vi "contorno prueba.vi"() -> ()   [LabVIEW 2020]
uses:
  <vilib>/userDefined/High Color/IMAQdx.ctl
  <vilib>/vision/Management.llb/Cast Image 2 Method.ctl
  <vilib>/vision/Contour.llb/IMAQ Connect Range Setting.ctl
  <vilib>/vision/Contour.llb/IMAQ Contour Curve Extraction.ctl
  <vilib>/vision/driver/NI_Vision_Acquisition_Software.lvlib
  <vilib>/vision/NI_Vision_Development_Module.lvlib
panel:
  out "Image 2":T1(plugin-control)
  in  "y":u8
  out "Image":T1(plugin-control)
  out "new picture":picture
  in  "Session In":T2="cam1"
  in  "stop":bool
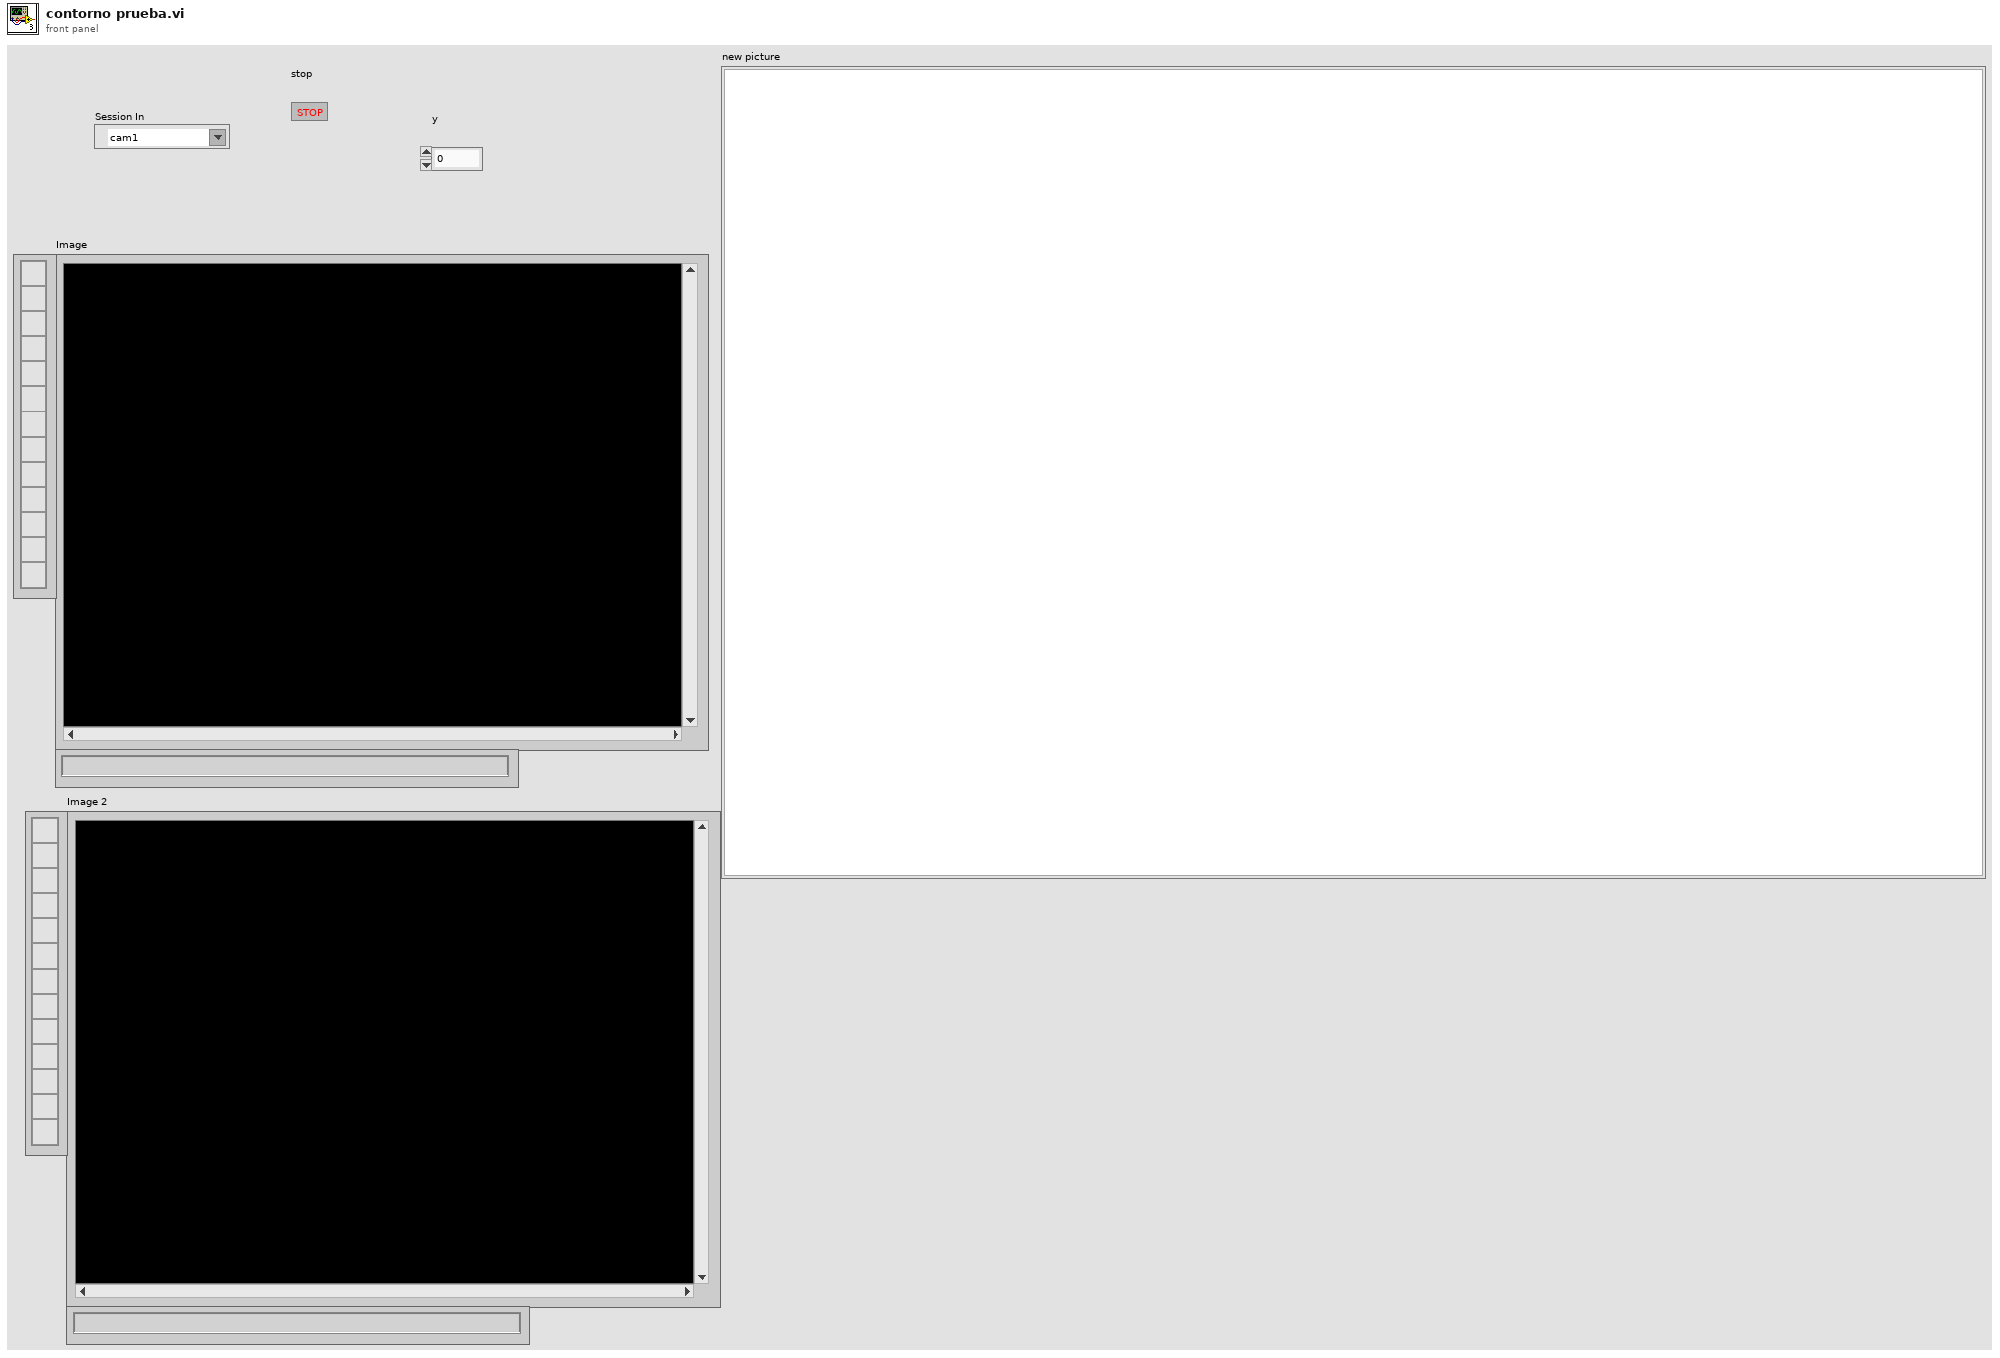
[diagram p1: front panel]
types:
  T1 = typedef "IMAQ Image.ctl" = refnum<image>
  T2 = typedef "IMAQdx.ctl" = refnum<k21>
  T3 = cluster{"Overlay?":bool, "Color":u32, "Width":u32, "Maintain Width?":bool}
  T4 = typedef "IMAQ Connect Range Setting.ctl" = cluster{"Match Constraints":u32, "Min":dbl, "Max":dbl}
  T5 = enum16{"Closest To Search Start", "Maximum Length", "Strongest Mean Gradient Change"}
  T6 = enum16{"Rect Left To Right", "Rect Right To Left", "Rect Top To Bottom", "Rect Bottom To Top", "Annulus Inner To Outer", "Annulus Outer To Inner", "Annulus Start Angle To End Angle", "Annulus End Angle To Start Angle"}
  T7 = typedef "IMAQ Contour Curve Extraction.ctl" = cluster{"Extraction Mode":u32, "Edge Threshold":i32, "Edge Filter Size":u32, "Min Length":i32, "Search Step Size":i32, "Max Endpoint Gap":i32, "Subpixel":bool}
  T8 = typedef "Image Type" = u32
  T9 = typedef "Cast Image 2 Method.ctl" = u32
  T10 = cluster{"Global Rectangle":i32[], "Contours":cluster{"Contour Type":u32, "ROI Type":u32, "Points":i32[]}[]}
  T11 = typedef "imagedata.ctl" = cluster{"image type":i32, "image depth":i32, "image":u8[], "mask":u8[], "colors":u32[], "Rectangle":cluster{"left":i16, "top":i16, "right":i16, "bottom":i16}}
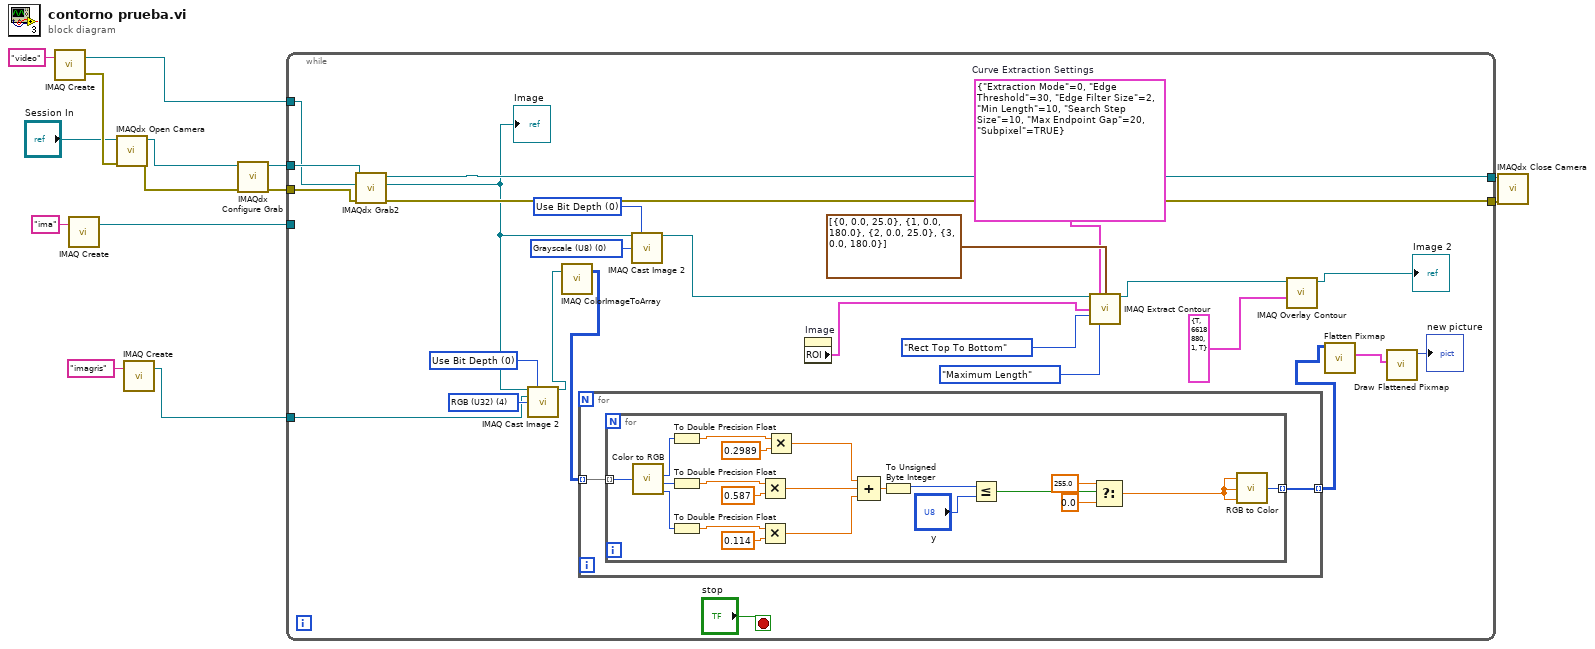
[diagram p0: block diagram]
diagram:
  n1 = call "IMAQ Create"("Image Name"="video") -> ("New Image"=w11:T1, "error out"=w14:errorcluster)  [unwired: 4 in]
  n2 = call "IMAQ Create"("Image Name"="ima") -> ("New Image"=w3:T1)  [unwired: 4 in, 1 out]
  n3 = call <vilib>:"IMAQdx Open Camera.vi"("error in"=w14, "Session In"="Session In") -> ("error out"=w7:errorcluster, "Session Out"=w13:T2)  [unwired: 8 in]
  n4 = call "IMAQ Create"("Image Name"="imagris") -> ("New Image"=w1:T1)  [unwired: 4 in, 1 out]
  n5 = call <vilib>:"IMAQdx Configure Grab.vi"("error in"=w7, "Session In"=w13) -> ("error out"=w8:errorcluster, "Session Out"=w12:T2)  [unwired: 8 in]
  n6 = while {
    tunnel: w12 -> [w40]
    tunnel: w11 -> [w39]
    tunnel: [w30] -> w10
    tunnel: [w29] -> w9
    tunnel: w8 -> [w37]
    tunnel: w3 -> [_]
    tunnel: w1 -> [w34]
    stop <- "stop" stop-if-true
    w20 = T7 {"Extraction Mode"=0, "Edge Threshold"=30, "Edge Filter Size"=2, "Min Length"=10, "Search Step Size"=10, "Max Endpoint Gap"=20, "Subpixel"=TRUE}  # Curve Extraction Settings
    w24 = T8 0 items=["Grayscale (U8)", "Grayscale (I16)", "Grayscale (SGL)", "Complex (CSG)", "RGB (U32)", "HSL (U32)", "RGB (U64)", "Grayscale (U16)"] ("Image Type")
    w25 = T9 0 items=["Use Bit Depth", "Shift", "Use Lookup Table"] ("Method")
    w35 = T9 0 items=["Use Bit Depth", "Shift", "Use Lookup Table"] ("Method")
    w36 = T8 4 items=["Grayscale (U8)", "Grayscale (I16)", "Grayscale (SGL)", "Complex (CSG)", "RGB (U32)", "HSL (U32)", "RGB (U64)", "Grayscale (U16)"] ("Image Type")
    n7 = call <vilib>:"IMAQdx Grab2.vi"("error in"=w37, "Image In"=w39, "Session In"=w40) -> ("error out"=w29:errorcluster, "Image Out"=w26:T1, "Session Out"=w30:T2)  [unwired: 5 in, 1 out]
    "Image" <- w26
    n8 = call "IMAQ Cast Image 2"("Image Src"=w26, "Method"=w35, "Image Dst"=w34, "Image Type"=w36) -> ("Image Dst Out"=w33:T1)  [unwired: 10 in, 1 out]
    n9 = call "IMAQ ColorImageToArray"("Image"=w33) -> ("Image Pixels (U32)"=w28:u32[][])  [unwired: 3 in, 2 out]
    n10 = for {
      tunnel: w28 -> [w42] mode=indexing
      tunnel: [w41] -> w27 mode=indexing
      n11 = for {
        tunnel: w42 -> [w63] mode=indexing
        tunnel: [w43] -> w41 mode=indexing
        n12 = call <vilib>:"Color to RGB.vi"("Color"=w63) -> ("R"=w62:u8, "G"=w61:u8, "B"=w60:u8)  [unwired: 1 out]
        n13 = To Double Precision Float(number=w62) -> (double precision float=w52:dbl)
        n14 = To Double Precision Float(number=w61) -> (double precision float=w51:dbl)
        n15 = To Double Precision Float(number=w60) -> (double precision float=w50:dbl)
        n16 = Multiply(x=w51, y=0.587) -> (x*y=w55:dbl)
        n17 = Multiply(x=w50, y=0.114) -> (x*y=w54:dbl)
        n18 = Multiply(x=w52, y=0.2989) -> (x*y=w56:dbl)
        n19 = Compound Arithmetic op=ADD(w56, w55, w54) -> (w53:dbl)
        n20 = To Unsigned Byte Integer(number=w53) -> (unsigned 8bit integer=w48:u8)
        n21 = Less Or Equal?(x=w48, y="y") -> (x <= y?=w47:bool)
        n22 = Select(t=255.0, s=w47, f=0.0) -> (s? t:f=w49:dbl)
        n23 = call <vilib>:"RGB to Color.vi"("B"=w49, "G"=w49, "R"=w49) -> ("Color"=w43:u32)
      }
    }
    n24 = call "IMAQ Cast Image 2"("Image Src"=w26, "Method"=w25, "Image Type"=w24) -> ("Image Dst Out"=w19:T1)  [unwired: 11 in, 1 out]
    n25 = property on="Image" class="ImageControl"() -> ("ROI"=w18:T10)  [unwired: 2 in, 2 out]
    n26 = call "IMAQ Extract Contour"("Source Image"=w19, "Curve Extraction"=w20, "ROI Descriptor"=w18, "Search Direction"=T6."Rect Top To Bottom", "Contour Selection"=T5."Maximum Length", "Curve Connection"=T4[] [{"Match Constraints"=0, "Min"=0.0, "Max"=25.0}, {"Match Constraints"=1, "Min"=0.0, "Max"=180.0}, {"Match Constraints"=2, "Min"=0.0, "Max"=25.0}, {"Match Constraints"=3, "Min"=0.0, "Max"=180.0}]) -> ("Source Image Out"=w16:T1)  [unwired: 2 in, 7 out]
    n27 = call "IMAQ Overlay Contour"("Contour Points Settings"=T3 {"Overlay?"=TRUE, "Color"=6618880, "Width"=1, "Maintain Width?"=TRUE}, "Image"=w16) -> ("Image Out"=→"Image 2":T1)  [unwired: 4 in, 5 out]
    n28 = call <vilib>:"Flatten Pixmap.vi"("24-bit pixmap"=w27) -> ("image data"=w32:T11)  [unwired: 10 in]
    n29 = call <vilib>:"Draw Flattened Pixmap.vi"("image data"=w32) -> ("new picture"=→"new picture":picture)  [unwired: 8 in]
  }
  n30 = call <vilib>:"IMAQdx Close Camera.vi"("error in"=w9, "Session In"=w10) -> ()  [unwired: 9 in, 1 out]
